vi "factorial of a num.vi"() -> ()   [LabVIEW 2025]
panel:
  out "factorial":dbl
  in  "input":dbl
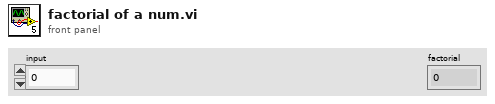
[diagram p1: front panel]
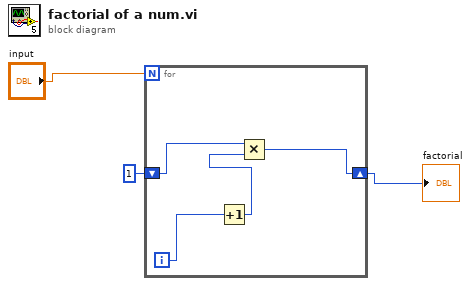
[diagram p0: block diagram]
diagram:
  n1 = for {
    N: "input" -> [_]
    shift-right: [w7] -> w2
    shift-left: 1 -> [w5]
    i -> [w6]
    n2 = Increment(x=w6) -> (x+1=w4:i32)
    n3 = Multiply(x=w5, y=w4) -> (x*y=w7:i32)
  }
  "factorial" <- w2
